vi "RGB_YUV.vi"(11 "Image In":T1) -> (3 "Image Out":T1)   [LabVIEW 2014]
uses:
  <vilib>/vision/Image Controls.llb/IMAQ Image.ctl
  <vilib>/Analysis/baseanly.llb/Real A x B.vi
  <vilib>/Analysis/Matrix/Numeric/Conversions/Array To Matrix - RA2.vi
  <vilib>/Analysis/Matrix/Numeric/Conversions/Matrix To Array - RM.vi
  <vilib>/Analysis/NI_AALBase.lvlib
  <vilib>/Analysis/Matrix/NI_Matrix.lvlib
  <vilib>/vision/NI_Vision_Development_Module.lvlib
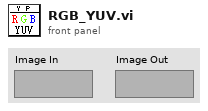
[diagram p1: front panel]
types:
  T1 = typedef "IMAQ Image.ctl" = refnum<image>
  T2 = typedef "Image Type" = u32
  T3 = cluster{"Red (or Hue) value":u8, "Green (or Sat) value":u8, "Blue (or Light or Val) value":u8}
  T4 = typedef "NI_Matrix.lvlib/RealMatrix.ctl" = dbl[][]
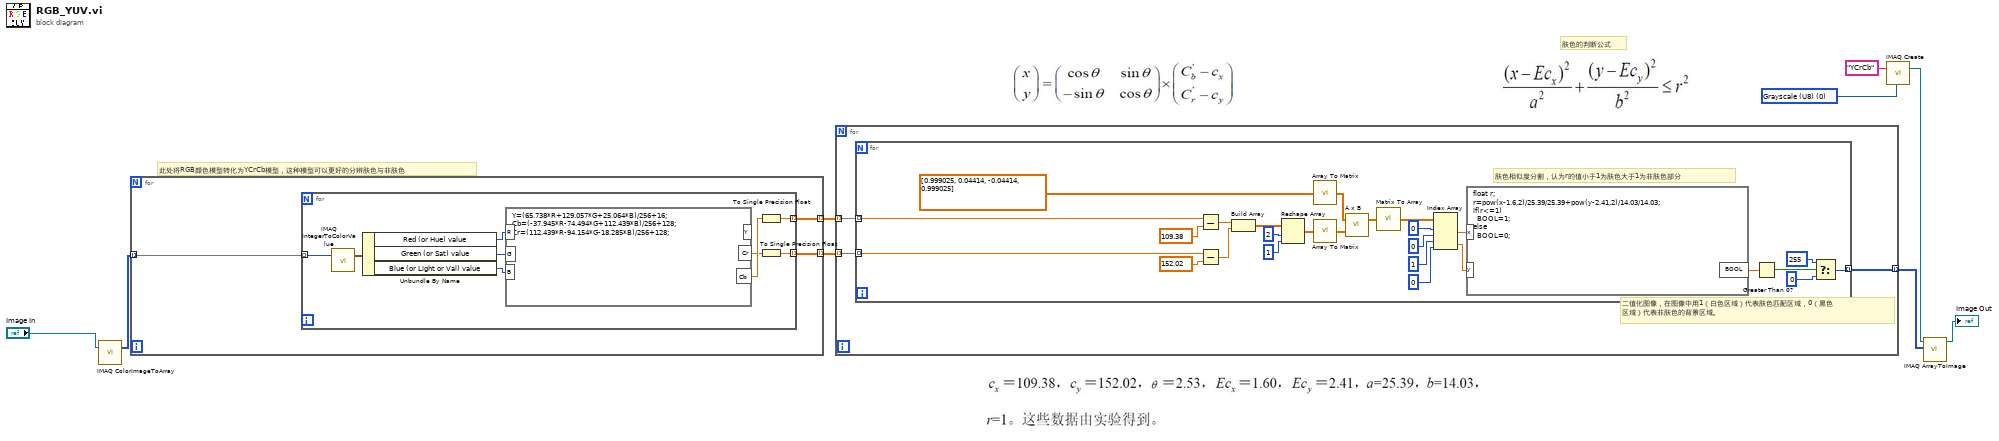
[diagram p0: block diagram]
diagram:
  w6 = T2 0 items=["Grayscale (U8)", "Grayscale (I16)", "Grayscale (SGL)", "Complex (CSG)", "RGB (U32)", "HSL (U32)", "RGB (U64)", "Grayscale (U16)"] ("Src")
  # "肤色的判断公式"
  # "此处将RGB颜色模型转化为YCrCb模型，这种模型可以更好的分辨肤色与非肤色"
  n1 = call "IMAQ ColorImageToArray"("Image"="Image In") -> ("Image Pixels (U32)"=w5:u32[][])  [unwired: 3 in, 2 out]
  n2 = for {
    tunnel: w5 -> [w12] mode=indexing
    tunnel: [w11] -> w8 mode=indexing
    tunnel: [w10] -> w9 mode=indexing
    n3 = for {
      tunnel: w12 -> [w17] mode=indexing
      tunnel: [w18] -> w11 mode=indexing
      tunnel: [w21] -> w10 mode=indexing
      n4 = call "IMAQ IntegerToColorValue"("U32 value"=w17) -> ("Color Value"=w16:T3)  [unwired: 4 in, 3 out]
      n5 = Unbundle By Name(w16) -> ("Red (or Hue) value"=w15:u8, "Green (or Sat) value"=w14:u8, "Blue (or Light or Val) value"=w13:u8)
      n6 = formula code="Y=(65.738*R+129.057*G+25.064*B)/256+16;\nCb=(-37.945*R-74.494*G+112.439*B)/256+128;\nCr=(112.439*R-94.154*G-18.285*B)/256+128;"("R"=w15, "G"=w14, "B"=w13) -> ("Cr"=w19:dbl, "Cb"=w20:dbl)  [unwired: 1 out]
      n7 = To Single Precision Float(number=w20) -> (single precision float=w21:sgl)
      n8 = To Single Precision Float(number=w19) -> (single precision float=w18:sgl)
    }
  }
  n9 = for {
    tunnel: w9 -> [w24] mode=indexing
    tunnel: w8 -> [w23] mode=indexing
    tunnel: [w22] -> w4 mode=indexing
    # "二值化图像，在图像中用1（白色区域）代表肤色匹配区域，0（黑色\n区域）代表非肤色的背景区域。"
    n10 = for {
      tunnel: w24 -> [w32] mode=indexing
      tunnel: w23 -> [w31] mode=indexing
      tunnel: [w27] -> w22 mode=indexing
      # "肤色相似度分割，认为r的值小于1为肤色大于1为非肤色部分"
      n11 = Subtract(x=w32, y=109.38) -> (x-y=w48:dbl)
      n12 = Subtract(x=w31, y=152.02) -> (x-y=w47:dbl)
      n13 = Build Array(w48, w47) -> (w43:dbl[])
      n14 = Reshape Array(w43, 2 ("维数大小"), 1 ("维数大小")) -> (w40:dbl[][])
      n15 = call-poly <vilib>:"Array To Matrix.vi"("Real 2D Array"=dbl[][] [[0.999025, 0.04414], [-0.04414, 0.999025]]) -> ("Real Matrix"=w46:T4)
      n16 = call-poly <vilib>:"Array To Matrix.vi"("Real 2D Array"=w40) -> ("Real Matrix"=w45:T4)
      n17 = call-poly <vilib>:"A x B.vi"("B"=w45, "A"=w46) -> ("A x B"=w44:T4)  [unwired: 1 out]
      n18 = call-poly <vilib>:"Matrix To Array.vi"("Real Matrix"=w44) -> ("Real 2D Array"=w38:dbl[][])
      n19 = Index Array(array=w38, index (row) #1=0 ("索引"), index (col) #1=0 ("索引"), index (row) #2=1 ("索引"), index (col) #2=0 ("索引")) -> (element #1=w34:dbl, element #2=w33:dbl)
      n20 = formula code="float r;\nr=pow(x-1.6,2)/25.39/25.39+pow(y-2.41,2)/14.03/14.03;\nif(r<=1)\n  BOOL=1;\nelse\n  BOOL=0;"("x"=w34, "y"=w33) -> ("BOOL"=w30:dbl)
      n21 = Greater Than 0?(x=w30) -> (x > 0?=w28:bool)
      n22 = Select(t=u8 255, s=w28, f=u8 0) -> (s? t:f=w27:u8)
    }
  }
  n23 = call "IMAQ Create"("Image Name"="YCrCb", "Image Type"=w6) -> ("New Image"=w3:T1)  [unwired: 3 in, 1 out]
  n24 = call "IMAQ ArrayToImage"("Image Pixels (U8)"=w4, "Image"=w3) -> ("Image Out"=→"Image Out":T1)  [unwired: 8 in, 1 out]
